vi "Generate Grid.vi"(1 "XYZ Resolution":dbl[](array[numeric]), 2 "Workspace Scope":T1) -> (0 "grid points":dbl[][](array[numeric]))   [LabVIEW 2014, in "Delta Analyzor.lvclass"]
uses:
  Delta Analyzor.lvclass
  Workspace Scope.ctl
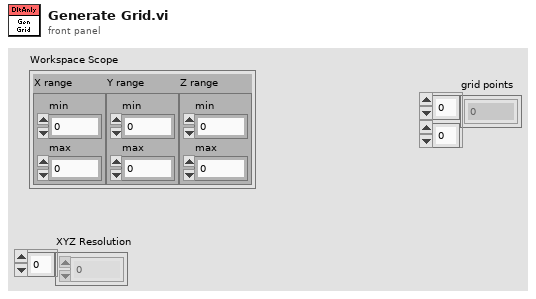
[diagram p1: front panel]
types:
  T1 = typedef "Delta Analyzor.lvclass/Workspace Scope.ctl" = cluster{"X range":cluster{"min":dbl, "max":dbl}, "Y range":cluster{"min":dbl, "max":dbl}, "Z range":cluster{"min":dbl, "max":dbl}}
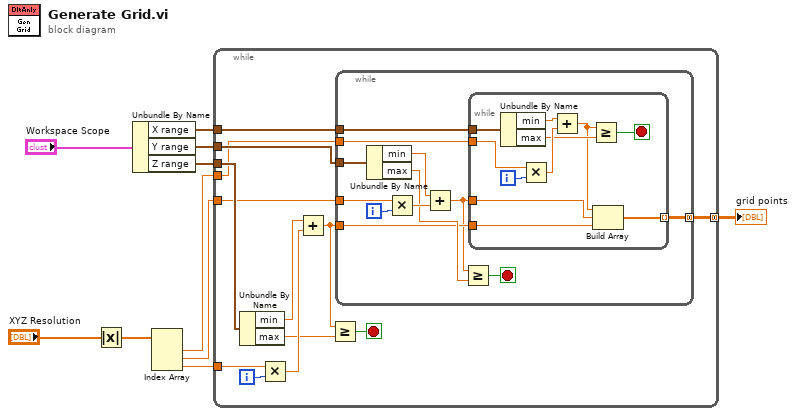
[diagram p0: block diagram]
diagram:
  n1 = Absolute Value(x="XYZ Resolution") -> (abs(x)=w8:dbl[])
  n2 = Unbundle By Name("Workspace Scope") -> ("X range"=w3:cluster{"min":dbl, "max":dbl}, "Y range"=w2:cluster{"min":dbl, "max":dbl}, "Z range"=w1:cluster{"min":dbl, "max":dbl})
  n3 = Index Array(array=w8) -> (element #1=w5:dbl, element #2=w6:dbl, element #3=w7:dbl)  [unwired: 3 in]
  n4 = while {
    tunnel: w1 -> [w18]
    tunnel: w7 -> [w17]
    tunnel: w2 -> [w16]
    tunnel: w6 -> [w15]
    tunnel: w3 -> [w14]
    tunnel: w5 -> [w13]
    tunnel: [w11] -> w4 mode=concatenating
    i -> [w22]
    stop <- w19 stop-if-true
    n5 = Unbundle By Name(w18) -> ("min"=w23:dbl, "max"=w20:dbl)
    n6 = Multiply(x=w17, y=w22) -> (x*y=w21:dbl)
    n7 = Add(x=w23, y=w21) -> (x+y=w12:dbl)
    n8 = Greater Or Equal?(x=w12, y=w20) -> (x >= y?=w19:bool)
    n9 = while {
      tunnel: w16 -> [w33]
      tunnel: w15 -> [w31]
      tunnel: w14 -> [w28]
      tunnel: w13 -> [w27]
      tunnel: w12 -> [w26]
      tunnel: [w24] -> w11 mode=concatenating
      i -> [w32]
      stop <- w29 stop-if-true
      n10 = Unbundle By Name(w33) -> ("min"=w34:dbl, "max"=w30:dbl)
      n11 = Multiply(x=w31, y=w32) -> (x*y=w35:dbl)
      n12 = Add(x=w34, y=w35) -> (x+y=w25:dbl)
      n13 = Greater Or Equal?(x=w25, y=w30) -> (x >= y?=w29:bool)
      n14 = while {
        tunnel: w28 -> [w45]
        tunnel: w27 -> [w43]
        tunnel: w26 -> [w37]
        tunnel: w25 -> [w38]
        tunnel: [w36] -> w24 mode=indexing
        i -> [w44]
        stop <- w40 stop-if-true
        n15 = Unbundle By Name(w45) -> ("min"=w46:dbl, "max"=w41:dbl)
        n16 = Multiply(x=w43, y=w44) -> (x*y=w42:dbl)
        n17 = Add(x=w46, y=w42) -> (x+y=w39:dbl)
        n18 = Greater Or Equal?(x=w39, y=w41) -> (x >= y?=w40:bool)
        n19 = Build Array(w39, w38, w37) -> (w36:dbl[])
      }
    }
  }
  "grid points" <- w4
